vi "DSF.Engine.Transceiver.Shutdown.vi"(8 "error in (no error)":errorcluster, 11 "GE Reflective Memory Transceiver in":refnum<class "DSF.Transceiver.GE Reflective Memory.lvclass">) -> (0 "error out":errorcluster, 3 "GE Reflective Memory Transceiver out":refnum<class "DSF.Transceiver.GE Reflective Memory.lvclass">)   [LabVIEW 2017, in "DSF.Transceiver.GE Reflective Memory.lvlib" / "DSF.Transceiver.GE Reflective Memory.lvclass"]
uses:
  DSF.Transceiver.GE Reflective Memory.lvclass
  DSF.Transceiver.GE Reflective Memory.lvclass/DSF.Transceiver.GE Reflective Memory.ctl
  <vilib>/NI/GE Reflective Memory Driver/GE 5565PIORC.lvclass/GE 5565PIORC.ctl
  <vilib>/NI/GE Reflective Memory Driver/Methods/GE 5565PIORC.DMA.Get Transfer Components (Block).vi
  <vilib>/NI/GE Reflective Memory Driver/GE 5565PIORC.lvclass
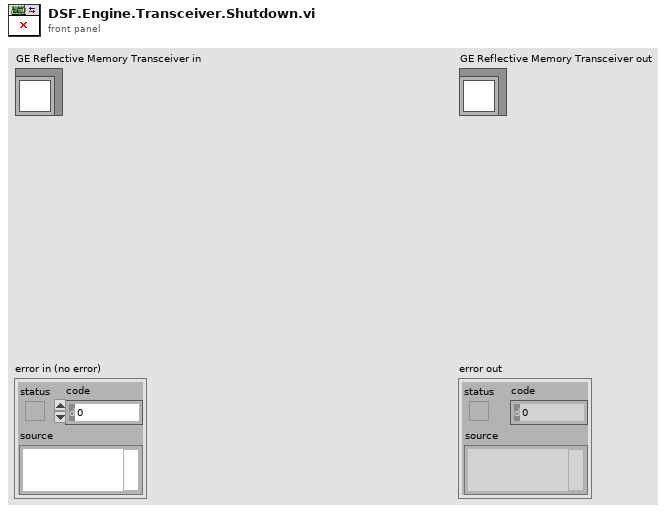
[diagram p1: front panel]
types:
  T1 = typedef "DSF.Transceiver.GE Reflective Memory.lvlib/DSF.Transceiver.GE Reflective Memory.lvclass/DSF.Transceiver.GE Reflective Memory.Transfer Group Parameters.ctl" = cluster{"DMA Transfer Specs":T2[]}
  T2 = typedef "GE 5565PIORC.lvclass/GE 5565PIORC.Typedef.DMA Transfer Spec.ctl" = cluster{"RFM offset":u32, "Block Descriptors":T3[]}
  T3 = typedef "GE 5565PIORC.lvclass/GE 5565PIORC.Typedef.DMA Block Descriptor.ctl" = cluster{"descriptor ptr (VISA)":u32, "descriptor ptr (RFM)":u32, "descriptor size":u32, "descriptor params":T4}
  T4 = typedef "GE 5565PIORC.lvclass/GE 5565PIORC.Typedef.DMA Block Descriptor Params.ctl" = cluster{"data ptr (lower)":u32, "data ptr (upper)":u32, "data size":u32, "next descriptor ptr":u32}
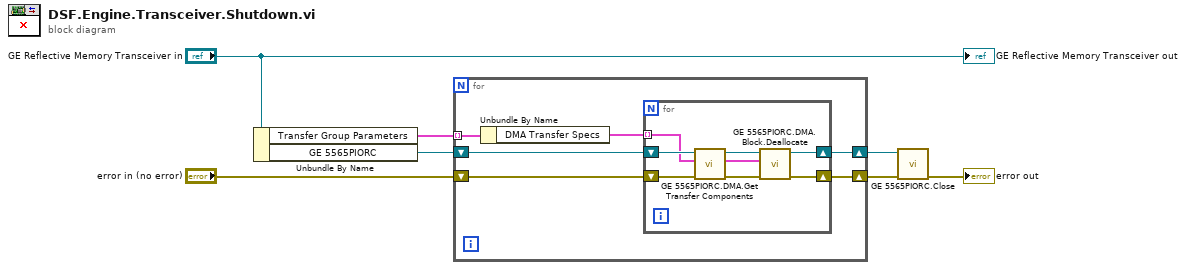
[diagram p0: block diagram]
diagram:
  n1 = Unbundle By Name("GE Reflective Memory Transceiver in") -> ("Transfer Group Parameters"=w7:T1[], "GE 5565PIORC"=w5:refnum<class "GE 5565PIORC.lvclass">)
  n2 = for {
    tunnel: w7 -> [w13] mode=indexing
    shift-right: [w9] -> w4
    shift-left: "error in (no error)" -> [w11]
    shift-right: [w8] -> w3
    shift-left: w5 -> [w10]
    n3 = Unbundle By Name(w13) -> ("DMA Transfer Specs"=w12:T2[])
    n4 = for {
      tunnel: w12 -> [w19] mode=indexing
      shift-right: [w16] -> w8
      shift-left: w10 -> [w20]
      shift-right: [w14] -> w9
      shift-left: w11 -> [w21]
      n5 = call-poly <vilib>:"GE 5565PIORC.DMA.Get Transfer Components.vi"("error in (no error)"=w21, "DMA Transfer Spec in"=w19, "GE 5565PIORC in"=w20) -> ("error out"=w15:errorcluster, "Block Descriptor"=w18:T3, "GE 5565PIORC out"=w17:refnum<class "GE 5565PIORC.lvclass">)  [unwired: 5 in, 1 out]
      n6 = call <vilib>:"GE 5565PIORC.DMA.Block.Deallocate.vi"("error in (no error)"=w15, "Block Descriptor"=w18, "GE 5565PIORC in"=w17) -> ("error out"=w14:errorcluster, "GE 5565PIORC out"=w16:refnum<class "GE 5565PIORC.lvclass">)  [unwired: 7 in]
    }
  }
  n7 = call <vilib>:"GE 5565PIORC.Close.vi"("error in (no error)"=w4, "GE 5565PIORC in"=w3) -> ("error out"=→"error out":errorcluster)  [unwired: 8 in, 1 out]
  "GE Reflective Memory Transceiver out" <- "GE Reflective Memory Transceiver in"
